vi "Spec Calculation.vi"(6 "기준값 열번호":i32, 7 "0기준?":bool, 9 "Resolution":string[][](array[string]), 10 "Condition in":string[][](array[string]), 11 "Spec Default":string[][](array[string])) -> (1 "Spec (DBL)":dbl[][](array[numeric]), 3 "Spec out":string[][](array[string]))   [LabVIEW 2020]
panel:
  out "error out":errorcluster caption="에러 출력"
  in  "error in":errorcluster caption="에러 입력(에러 없음)"
  # "0 : FUNC\n1 : FUNC_EXT\n2 : FUNC_CON\n3 : C1_VAL\n4 : C1_UNIT\n5 : RANGE_VAL\n6 : RANGE_UNIT"
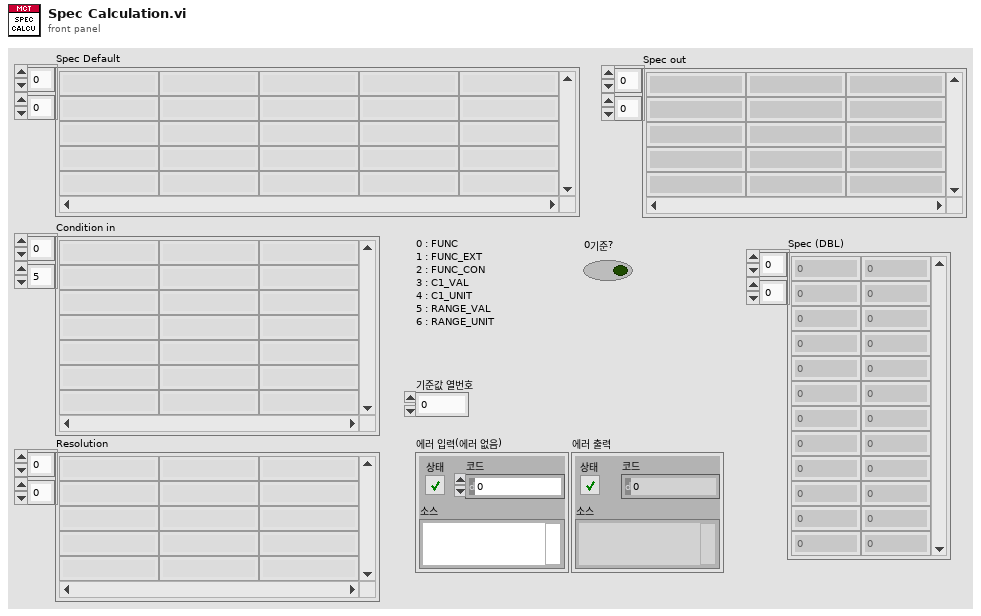
[diagram p1: front panel]
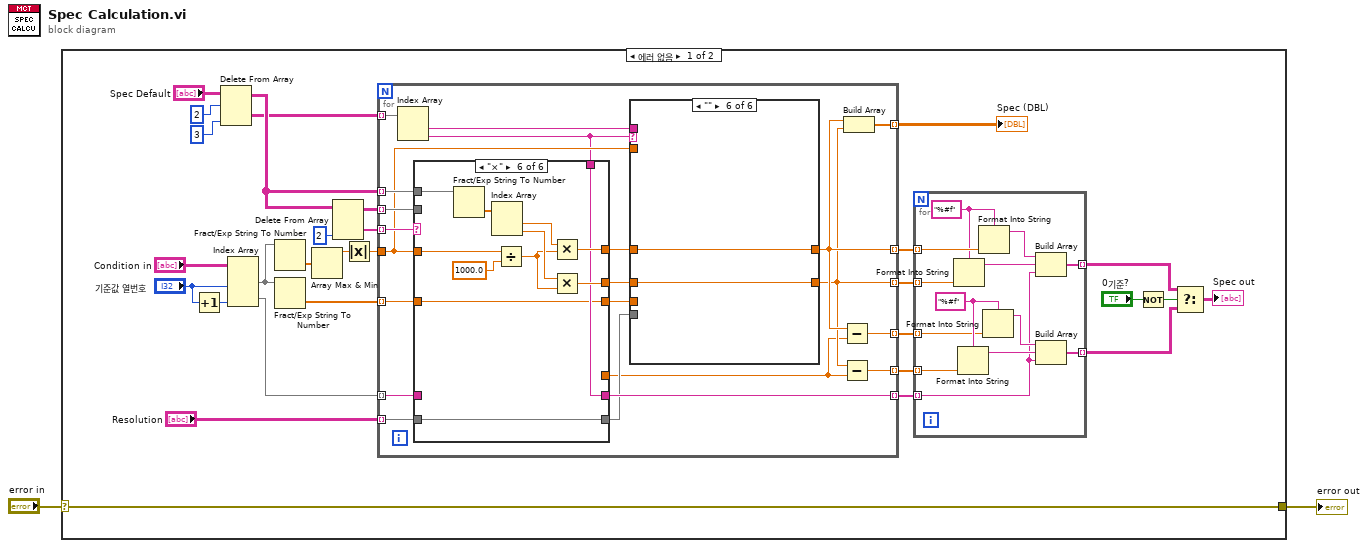
[diagram p0: block diagram]
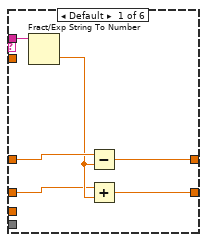
[diagram p2: hidden frame]
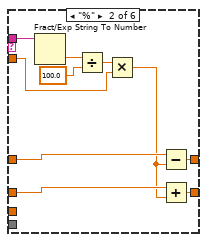
[diagram p3: hidden frame]
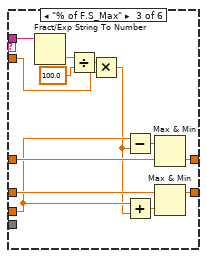
[diagram p4: hidden frame]
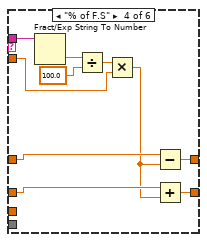
[diagram p5: hidden frame]
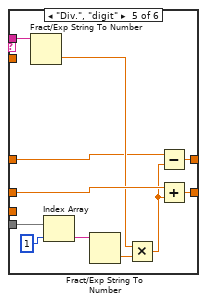
[diagram p6: hidden frame]
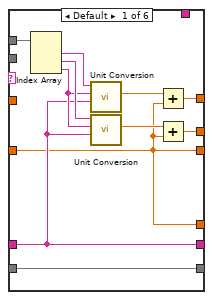
[diagram p7: hidden frame]
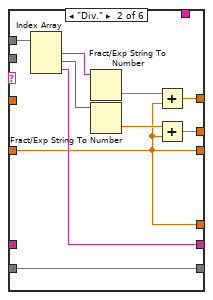
[diagram p8: hidden frame]
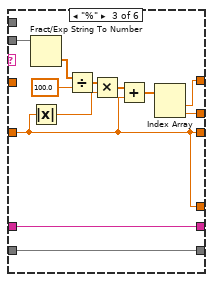
[diagram p9: hidden frame]
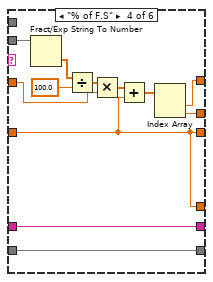
[diagram p10: hidden frame]
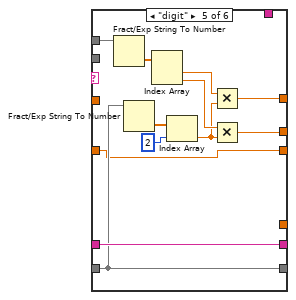
[diagram p11: hidden frame]
diagram:
  n1 = case shown="에러 없음" "error in" {
    selector: "error in" -> [w30 w188]
    tunnel: [w30 w188] -> w1
    frame No Error {
      n2 = Increment(x="기준값 열번호") -> (x+1=w8:i32)
      n3 = Delete From Array(array="Spec Default", length=2 ("길이"), index (col)=3 ("비활성화된 인덱스 (열)")) -> (deleted portion=w16:string[][], array with subset deleted=w17:string[][])  [unwired: 1 in]
      n4 = Index Array(array="Condition in", index (col) #1="기준값 열번호", index (col) #2=w8) -> (element #1=w13:string[], element #2=w25:string[])  [unwired: 2 in]
      n5 = Fract/Exp String To Number(string=w13) -> (number=w24:dbl[])  [unwired: 3 in, 1 out]
      n6 = Fract/Exp String To Number(string=w13) -> (number=w12:dbl[])  [unwired: 3 in, 1 out]
      n7 = Array Max & Min(array=w24) -> (max value=w23:dbl)  [unwired: 3 out]
      n8 = Delete From Array(array=w17, index (col)=2 ("비활성화된 인덱스 (열)")) -> (deleted portion=w32:string[], array with subset deleted=w28:string[][])  [unwired: 2 in]
      n9 = Absolute Value(x=w23) -> (abs(x)=w15:dbl)
      n10 = for {
        tunnel: w28 -> [w66] mode=indexing
        tunnel: w25 -> [w62] mode=indexing
        tunnel: w32 -> [w65] mode=indexing
        tunnel: w17 -> [w64] mode=indexing
        tunnel: [w54] -> w27 mode=indexing
        tunnel: [w53] -> w26 mode=indexing
        tunnel: w15 -> [w57]
        tunnel: [w63] -> w22 mode=indexing
        tunnel: "Resolution" -> [w50] mode=indexing
        tunnel: w16 -> [w61] mode=indexing
        tunnel: [w56] -> w14 mode=indexing
        tunnel: w12 -> [w55] mode=indexing
        tunnel: [w52] -> w11 mode=indexing
        tunnel: [w51] -> w10 mode=indexing
        n11 = Index Array(array=w61) -> (element #1=w60:string, element #2=w48:string)  [unwired: 2 in]
        n12 = case shown="\"×\"" w65 {
          tunnel: w66 -> [_ _ w151 w163 _ _]
          tunnel: w55 -> [w119 w130 w140 w152 w164 w179]
          tunnel: w64 -> [w129 w139 _ _ w174 w187]
          tunnel: w62 -> [w123 _ w142 w154 w175 _]
          tunnel: [w127 w138 w144 w156 w167 w183] -> w59
          tunnel: [w126 w137 w143 w155 w166 w182] -> w58
          tunnel: w57 -> [_ _ _ w157 _ w178]
          tunnel: [w123 w132 w142 w154 w175 w180] -> w63
          tunnel: w50 -> [w120 w131 w141 w153 w165 w181]
          tunnel: [w119 w130 w140 w152 _ _] -> w47
          tunnel: [w120 w131 w141 w153 w165 w181] -> w49
          tunnel: w48 -> [_ _ _ _ _ w180]
          tunnel: [w119 w130 w140 w152 w164 w179] -> w46
          frame Default {
            n13 = Index Array(array=w129) -> (element #1=w128:string, element #2=w125:string, element #3=w124:string)  [unwired: 3 in]
            n14 = call "Unit Conversion.vi"("환산단위"=w123, "입력단위"=w124, "입력값"=w128) -> ("환산값 (DBL)"=w122:dbl)  [unwired: 3 in, 5 out]
            n15 = call "Unit Conversion.vi"("환산단위"=w123, "입력단위"=w124, "입력값"=w125) -> ("환산값 (DBL)"=w121:dbl)  [unwired: 3 in, 5 out]
            n16 = Add(x=w122, y=w119) -> (x+y=w127:dbl)
            n17 = Add(x=w121, y=w119) -> (x+y=w126:dbl)
          }
          frame "Div." {
            n18 = Index Array(array=w139) -> (element #1=w136:string, element #2=w133:string, element #3=w132:string)  [unwired: 3 in]
            n19 = Fract/Exp String To Number(string=w136) -> (number=w135:dbl)  [unwired: 3 in, 1 out]
            n20 = Fract/Exp String To Number(string=w133) -> (number=w134:dbl)  [unwired: 3 in, 1 out]
            n21 = Add(x=w135, y=w130) -> (x+y=w138:dbl)
            n22 = Add(x=w134, y=w130) -> (x+y=w137:dbl)
          }
          frame "%" {
            n23 = Fract/Exp String To Number(string=w151) -> (number=w149:dbl[])  [unwired: 3 in, 1 out]
            n24 = Absolute Value(x=w140) -> (abs(x)=w145:dbl)
            n25 = Divide(x=w149, y=100.0) -> (x/y=w146:dbl[])
            n26 = Multiply(x=w146, y=w145) -> (x*y=w148:dbl[])
            n27 = Add(x=w148, y=w140) -> (x+y=w147:dbl[])
            n28 = Index Array(array=w147) -> (element #1=w144:dbl, element #2=w143:dbl)  [unwired: 2 in]
          }
          frame "% of F.S" {
            n29 = Fract/Exp String To Number(string=w163) -> (number=w161:dbl[])  [unwired: 3 in, 1 out]
            n30 = Divide(x=w161, y=100.0) -> (x/y=w158:dbl[])
            n31 = Multiply(x=w158, y=w157) -> (x*y=w160:dbl[])
            n32 = Add(x=w160, y=w152) -> (x+y=w159:dbl[])
            n33 = Index Array(array=w159) -> (element #1=w156:dbl, element #2=w155:dbl)  [unwired: 2 in]
          }
          frame "digit" {
            n34 = Fract/Exp String To Number(string=w174) -> (number=w173:dbl[])  [unwired: 3 in, 1 out]
            n35 = Fract/Exp String To Number(string=w165) -> (number=w171:dbl[])  [unwired: 3 in, 1 out]
            n36 = Index Array(array=w173) -> (element #1=w172:dbl, element #2=w169:dbl)  [unwired: 2 in]
            n37 = Index Array(array=w171, index=2 ("인덱스")) -> (element=w168:dbl)
            n38 = Multiply(x=w172, y=w168) -> (x*y=w167:dbl)
            n39 = Multiply(x=w169, y=w168) -> (x*y=w166:dbl)
          }
          frame "×" {
            n40 = Fract/Exp String To Number(string=w187) -> (number=w186:dbl[])  [unwired: 3 in, 1 out]
            n41 = Index Array(array=w186) -> (element #1=w185:dbl, element #2=w184:dbl)  [unwired: 2 in]
            n42 = Divide(x=w178, y=1000.0) -> (x/y=w176:dbl)
            n43 = Multiply(x=w185, y=w176) -> (x*y=w183:dbl)
            n44 = Multiply(x=w184, y=w176) -> (x*y=w182:dbl)
          }
        }
        n45 = case shown="\"\"" w48 {
          tunnel: [w72 w82 w83 w100 w116 w118] -> w54
          tunnel: [w71 w81 w90 w99 w115 w117] -> w53
          tunnel: w59 -> [w69 w80 w89 w98 w109 w118]
          tunnel: w60 -> [w70 w78 w95 w105 w113 _]
          tunnel: w58 -> [w67 w79 w88 w97 w114 w117]
          tunnel: w57 -> [_ w74 w91 w101 _ _]
          tunnel: w49 -> [_ _ _ _ w108 _]
          tunnel: w46 -> [_ _ w85 _ _ _]
          frame Default {
            n46 = Fract/Exp String To Number(string=w70) -> (number=w68:dbl)  [unwired: 3 in, 1 out]
            n47 = Subtract(x=w69, y=w68) -> (x-y=w72:dbl)
            n48 = Add(x=w67, y=w68) -> (x+y=w71:dbl)
          }
          frame "%" {
            n49 = Fract/Exp String To Number(string=w78) -> (number=w77:dbl)  [unwired: 3 in, 1 out]
            n50 = Divide(x=w77, y=100.0) -> (x/y=w75:dbl)
            n51 = Multiply(x=w75, y=w74) -> (x*y=w73:dbl)
            n52 = Subtract(x=w80, y=w73) -> (x-y=w82:dbl)
            n53 = Add(x=w79, y=w73) -> (x+y=w81:dbl)
          }
          frame "% of F.S_Max" {
            n54 = Fract/Exp String To Number(string=w95) -> (number=w94:dbl)  [unwired: 3 in, 1 out]
            n55 = Divide(x=w94, y=100.0) -> (x/y=w92:dbl)
            n56 = Multiply(x=w92, y=w91) -> (x*y=w84:dbl)
            n57 = Subtract(x=w85, y=w84) -> (x-y=w86:dbl)
            n58 = Add(x=w85, y=w84) -> (x+y=w87:dbl)
            n59 = Max & Min(x=w86, y=w89) -> (min(x,y)=w83:dbl)  [unwired: 1 out]
            n60 = Max & Min(x=w88, y=w87) -> (max(x,y)=w90:dbl)  [unwired: 1 out]
          }
          frame "% of F.S" {
            n61 = Fract/Exp String To Number(string=w105) -> (number=w104:dbl)  [unwired: 3 in, 1 out]
            n62 = Divide(x=w104, y=100.0) -> (x/y=w102:dbl)
            n63 = Multiply(x=w102, y=w101) -> (x*y=w96:dbl)
            n64 = Subtract(x=w98, y=w96) -> (x-y=w100:dbl)
            n65 = Add(x=w97, y=w96) -> (x+y=w99:dbl)
          }
          frame "Div.", "digit" {
            n66 = Fract/Exp String To Number(string=w113) -> (number=w112:dbl)  [unwired: 3 in, 1 out]
            n67 = Index Array(array=w108, index=1 ("인덱스")) -> (element=w106:string)
            n68 = Fract/Exp String To Number(string=w106) -> (number=w111:dbl)  [unwired: 3 in, 1 out]
            n69 = Multiply(x=w112, y=w111) -> (x*y=w110:dbl)
            n70 = Subtract(x=w109, y=w110) -> (x-y=w116:dbl)
            n71 = Add(x=w114, y=w110) -> (x+y=w115:dbl)
          }
          frame "" {
          }
        }
        n72 = Subtract(x=w54, y=w47) -> (x-y=w52:dbl)
        n73 = Subtract(x=w53, y=w47) -> (x-y=w51:dbl)
        n74 = Build Array(w54, w53) -> (w56:dbl[])
      }
      "Spec (DBL)" <- w14
      n75 = for {
        tunnel: w27 -> [w44] mode=indexing
        tunnel: w26 -> [w40] mode=indexing
        tunnel: w22 -> [w34] mode=indexing
        tunnel: [w45] -> w6 mode=indexing
        tunnel: w11 -> [w36] mode=indexing
        tunnel: w10 -> [w35] mode=indexing
        tunnel: [w33] -> w5 mode=indexing
        w38 = "%#f" ("포맷 문자열")
        w42 = "%#f" ("포맷 문자열")
        n76 = Format Into String(format string=w42, w40) -> (resulting string=w41:string)  [unwired: 2 in, 1 out]
        n77 = Format Into String(format string=w38, w35) -> (resulting string=w39:string)  [unwired: 2 in, 1 out]
        n78 = Format Into String(format string=w42, w44) -> (resulting string=w43:string)  [unwired: 2 in, 1 out]
        n79 = Format Into String(format string=w38, w36) -> (resulting string=w37:string)  [unwired: 2 in, 1 out]
        n80 = Build Array(w43, w41, w34) -> (w45:string[])
        n81 = Build Array(w37, w39, w34) -> (w33:string[])
      }
      n82 = Not(x="0기준?") -> (.not. x?=w3:bool)
      n83 = Select(t=w6, s=w3, f=w5) -> (s? t:f=→"Spec out":string[][])
    }
    frame Error {
    }
  }
  "error out" <- w1
